vi "4145 Check ON LINE.vi"(8 "error in (no error)":errorcluster, 11 "4145_GPIB_COM_IN":T1={"Address_string"="17", "timeout ms"=25000, "Terminator"=",", "LoggerQueue"=refnum}) -> (0 "error out":errorcluster, 1 "GPIB error":i16, 2 "on line?":bool, 3 "4145_GPIB_COM_OUT":T1={"Address_string"="17", "timeout ms"=25000, "Terminator"=",", "LoggerQueue"=refnum})   [LabVIEW 2014]
uses:
  typedef/4145_GPIB_Com.ctl
  typedef/4145_que_msg.ctl
  typedef/4145 command enum.ctl
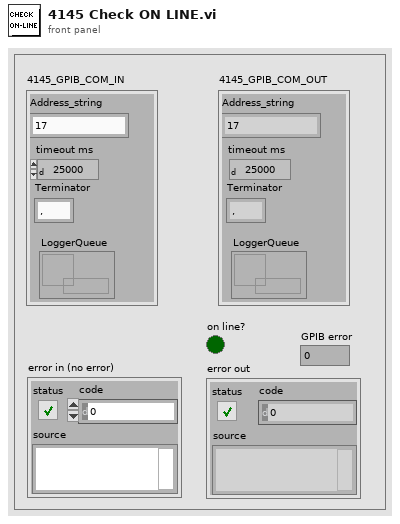
[diagram p1: front panel]
types:
  T1 = typedef "4145_GPIB_Com.ctl" = cluster{"Address_string":string, "timeout ms":u32, "Terminator":string, "LoggerQueue":refnum<queue>}
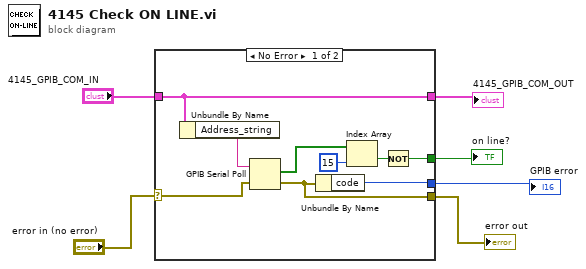
[diagram p0: block diagram]
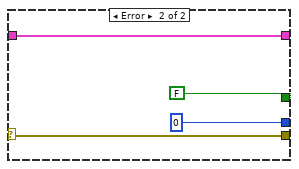
[diagram p2: hidden frame]
diagram:
  n1 = case shown="No Error" "error in (no error)" {
    selector: "error in (no error)" -> [w11 w19]
    tunnel: [w7 w19] -> w5
    tunnel: "4145_GPIB_COM_IN" -> [w15 w18]
    tunnel: [w15 w18] -> w3
    tunnel: [w13 FALSE] -> w2
    tunnel: [w8 i16 0 ("GPIB error")] -> w1
    frame No Error {
      n2 = Unbundle By Name(w15) -> ("Address_string"=w12:string)
      n3 = GPIB Serial Poll(0:w12, 1:w11) -> (3:w10:bool[], 4:w7:errorcluster)  [unwired: 1 out]
      n4 = Unbundle By Name(w7) -> ("code"=w8:i32)
      n5 = Index Array(array=w10, index=15) -> (element=w9:bool)
      n6 = Not(x=w9) -> (.not. x?=w13:bool)
    }
    frame Error {
    }
  }
  "error out" <- w5
  "4145_GPIB_COM_OUT" <- w3
  "on line?" <- w2
  "GPIB error" <- w1
